vi "Collate Port Array.vi"(8 "error in (no error)":errorcluster, 10 "data":u32[][](array[numeric]), 11 "DAQmxDI in":refnum<class "DAQmxDI.lvclass">) -> (0 "error out":errorcluster, 2 "Waveforms":waveform(dbl)[](array[waveform]), 3 "DAQmxDI out":refnum<class "DAQmxDI.lvclass">)   [LabVIEW 2020, in "VolatusDAQ.lvlib" / "DAQmxDI.lvclass"]
uses:
  DAQmxDI.lvclass
  DAQmxDI.lvclass/DAQmxDI.ctl
  VolatusDAQ.lvlib
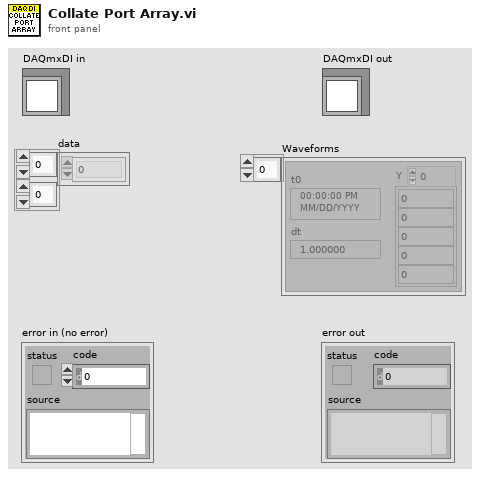
[diagram p1: front panel]
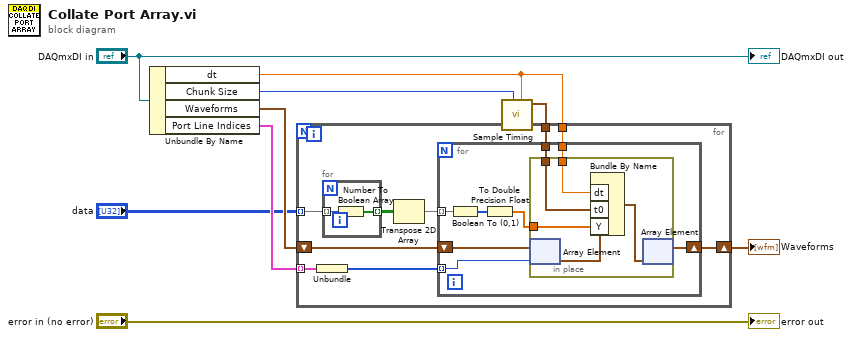
[diagram p0: block diagram]
diagram:
  n1 = Unbundle By Name("DAQmxDI in") -> ("dt"=w4:dbl, "Chunk Size"=w8:i32, "Waveforms"=w7:waveform(dbl)[], "Port Line Indices"=w6:cluster{"Channel Indices":i32[]}[])
  n2 = call "Sample Timing.vi"("dt"=w4, "# Samples"=w8) -> ("t0"=w5:timestamp)  [unwired: 8 in, 1 out]
  n3 = for {
    tunnel: "data" -> [w11] mode=indexing
    shift-right: [w13] -> w1
    shift-left: w7 -> [w17]
    tunnel: w6 -> [w18] mode=indexing
    tunnel: w5 -> [w15]
    tunnel: w4 -> [w14]
    n4 = Unbundle(w18) -> ("Channel Indices"=w16:i32[])
    n5 = for {
      tunnel: w11 -> [w20] mode=indexing
      tunnel: [w19] -> w12 mode=indexing
      n6 = Number To Boolean Array(number=w20) -> (Boolean array=w19:bool[])
    }
    n7 = Transpose 2D Array(2D array=w12) -> (transposed array=w10:bool[][])
    n8 = for {
      shift-right: [w24] -> w13
      shift-left: w17 -> [w28]
      tunnel: w16 -> [w27] mode=indexing
      tunnel: w15 -> [w26]
      tunnel: w14 -> [w25]
      tunnel: w10 -> [w23] mode=indexing
      n9 = Boolean To (0,1)(Boolean=w23) -> (0, 1=w22:i16[])
      n10 = To Double Precision Float(number=w22) -> (double precision float=w21:dbl[])
      n11 = in-place {
        in-place-border: w26 -> [w30]
        in-place-border: w25 -> [w32]
        in-place-border: w21 -> [w29]
        n12 = in-place-array #1(w28, w27) -> (w33:waveform(dbl))
        n13 = Bundle By Name(cluster=w33, "dt"=w32, "t0"=w30, "Y"=w29) -> (w31:waveform(dbl))
        n14 = in-place-array #1(w31) -> (w24:waveform(dbl)[])  [unwired: 1 out]
      }
    }
  }
  "Waveforms" <- w1
  "error out" <- "error in (no error)"
  "DAQmxDI out" <- "DAQmxDI in"
